vi "Login.vi"(1 "Password":string, 2 "Username":string) -> (0 "Signal":bool)   [LabVIEW 2024]
uses:
  <vilib>/Utility/file.llb/Read Delimited Spreadsheet (string).vi
panel:
  in  "Login":bool
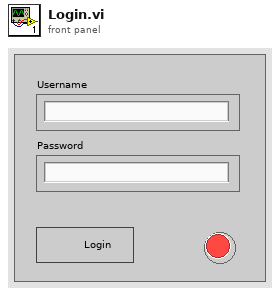
[diagram p1: front panel]
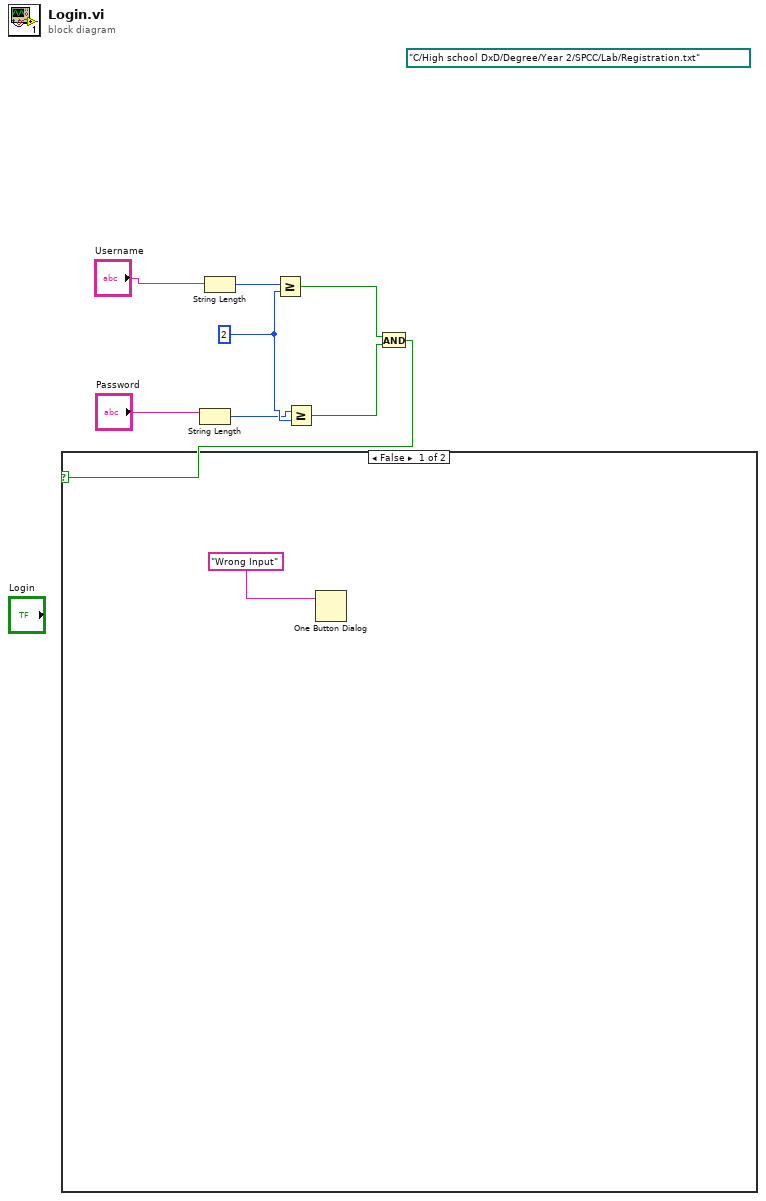
[diagram p0: block diagram]
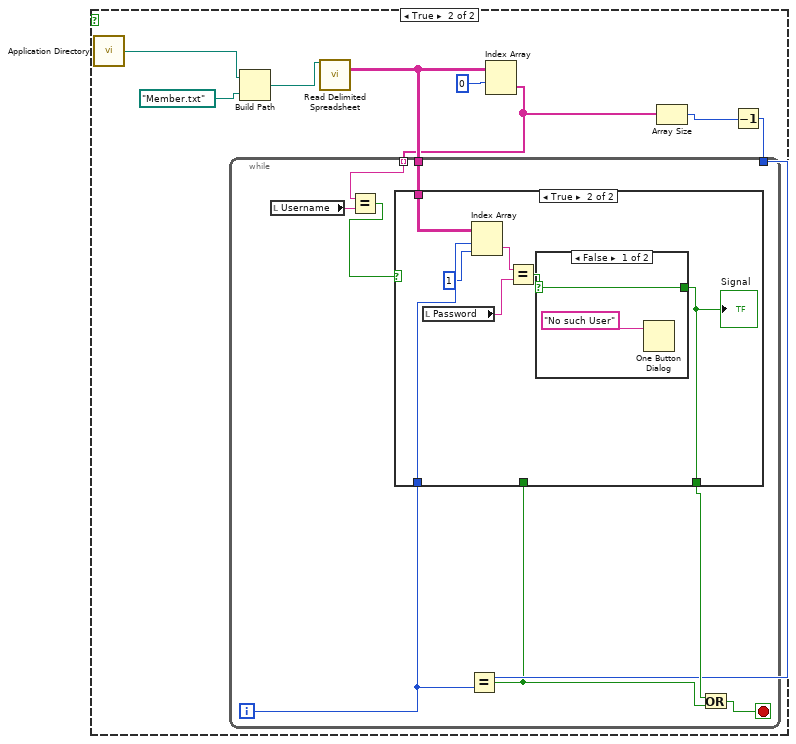
[diagram p2: hidden frame]
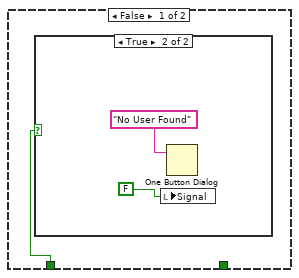
[diagram p3: hidden frame]
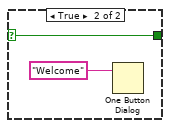
[diagram p5: hidden frame]
diagram:
  w2 = 2 ("length")
  (unwired) path "C:/High school DxD/Degree/Year 2/SPCC/Lab/Registration.txt" ("file path (dialog if empty)")
  n1 = String Length(string="Password") -> (length=w1:i32)
  n2 = String Length(string="Username") -> (length=w6:i32)
  n3 = Greater Or Equal?(x=w6, y=w2) -> (x >= y?=w4:bool)
  n4 = Greater Or Equal?(x=w1, y=w2) -> (x >= y?=w5:bool)
  n5 = And(x=w4, y=w5) -> (x .and. y?=w3:bool)
  n6 = case shown="False" w3 {
    frame False {
      n7 = One Button Dialog(message="Wrong Input") -> ()  [unwired: 1 in, 1 out]
    }
    frame True {
      n8 = call <vilib>:"Application Directory.vi"() -> ("Application Directory"=w14:path)
      n9 = Build Path(base path=w14, name or relative path=path "Member.txt") -> (appended path=w12:path)
      n10 = call-poly <vilib>:"Read Delimited Spreadsheet.vi"("file path (dialog if empty)"=w12) -> ("all rows"=w11:string[][])  [unwired: 9 in, 5 out]
      n11 = Index Array "Index Array"(array=w11, index (row)=0) -> (element=w10:string[])  [unwired: 1 in]
      n12 = Array Size(array=w10) -> (size(s)=w15:i32)
      n13 = Decrement(x=w15) -> (x-1=w16:i32)
      n14 = while {
        tunnel: w10 -> [w26] mode=indexing
        tunnel: [w21] -> _
        tunnel: w16 -> [w21]
        tunnel: w11 -> [w18]
        i -> [w20]
        stop <- w22 stop-if-true
        n15 = local read "Username"() -> (w25:string)
        n16 = Equal?(x=w26, y=w25) -> (x = y?=w24:bool)
        n17 = Equal?(x=w21, y=w20) -> (x = y?=w19:bool)
        n18 = case shown="True" w24 {
          tunnel: [_ w35] -> w23
          tunnel: w20 -> [_ w32]
          tunnel: w19 -> [w27 _]
          tunnel: w18 -> [_ w33]
          frame False {
            n19 = case shown="True" w27 {
              frame False {
              }
              frame True {
                n20 = local write "Signal"(FALSE ("Signal")) -> ()
                n21 = One Button Dialog(message="No User Found") -> ()  [unwired: 1 in, 1 out]
              }
            }
          }
          frame True {
            n22 = local read "Password"() -> (w36:string)
            n23 = Index Array "Index Array"(array=w33, index (row)=w32, index (col)=1 ("index")) -> (element=w30:string)
            n24 = Equal?(x=w30, y=w36) -> (x = y?=w34:bool)
            n25 = case shown="False" w34 {
              selector: w34 -> [w38 w40]
              tunnel: [w38 w40] -> w35
              frame False {
                n26 = One Button Dialog(message="No such User") -> ()  [unwired: 1 in, 1 out]
              }
              frame True {
                n27 = One Button Dialog(message="Welcome") -> ()  [unwired: 1 in, 1 out]
              }
            }
            "Signal" <- w35
          }
        }
        n28 = Or(x=w23, y=w19) -> (x .or. y?=w22:bool)
      }
    }
  }
